vi "CEID Manager.vi"(8 "error in (no error)":errorcluster, 11 "CEID Data":cluster{"CEID":u32, "RPTID":u32[]}[](array[cluster])) -> (0 "error out":errorcluster)   [LabVIEW 2020, in "SECS Scenarios.lvlib" / "34-CEID Setup.lvclass"]
uses:
  34-CEID Setup.lvclass
  SECS Communication/SECS Data Class/CEID Data.ctl
  SECS Communication/SECS Data Class/Remove CEID.vi
  SECS Communication/SECS Data Class/Add CEID.vi
  SECS Communication/SECS Data Class/Get All CEID Data.vi
  SECS Communication/SECS Data Class/SECS Data Class.lvclass
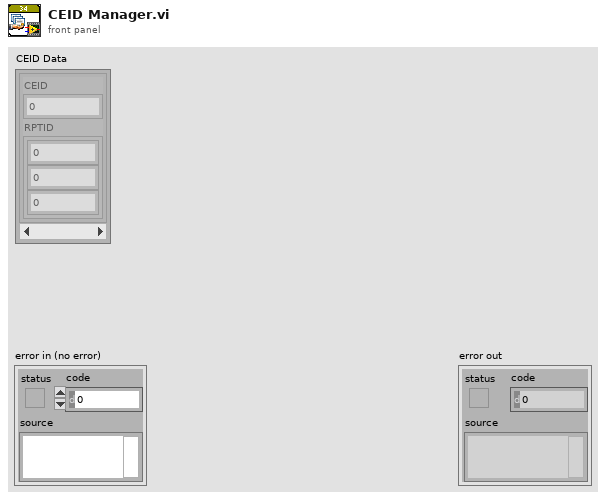
[diagram p1: front panel]
types:
  T1 = typedef "SECS Communication.lvlib/SECS Data Class.lvclass/CEID Data.ctl" = cluster{"Enable":bool, "CEID":u32, "Name":string, "Description":string, "RPTID":u32[], "Dynamic":bool}
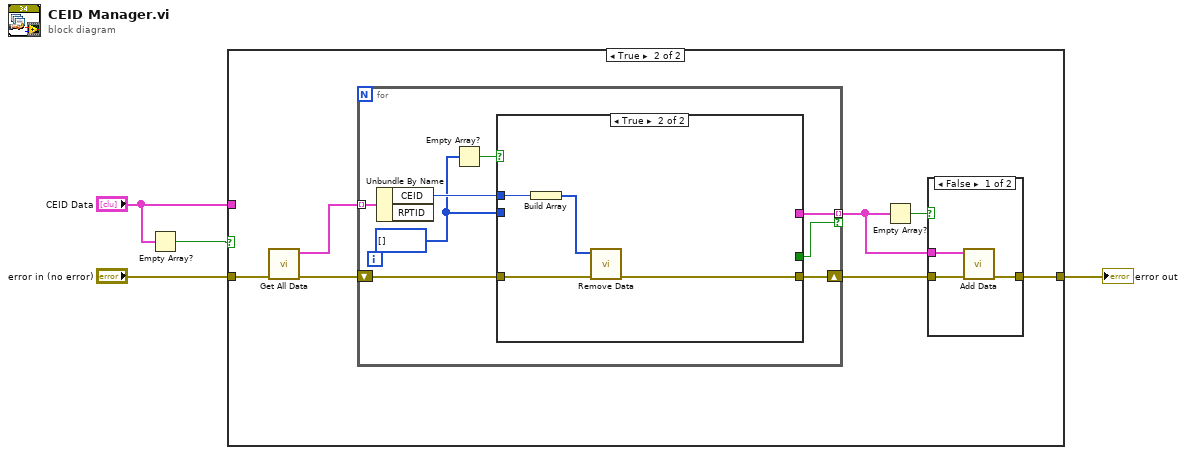
[diagram p0: block diagram]
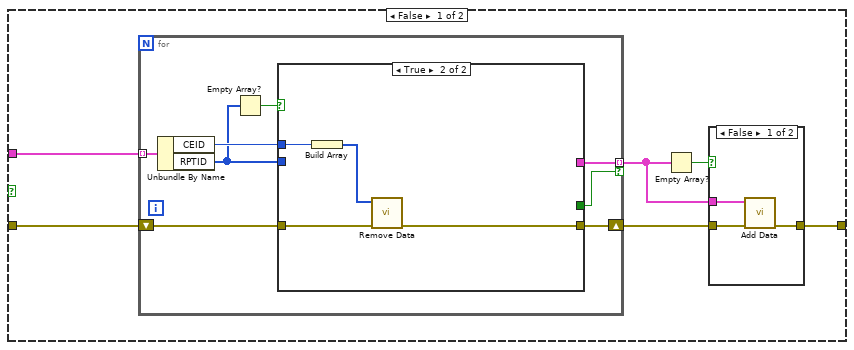
[diagram p2: hidden frame]
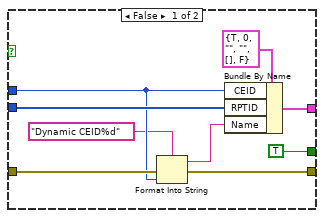
[diagram p4: hidden frame]
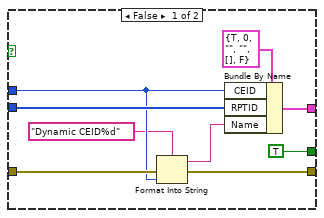
[diagram p6: hidden frame]
diagram:
  n1 = Empty Array?(array="CEID Data") -> (empty?=w1:bool)
  n2 = case shown="True" w1 {
    tunnel: "error in (no error)" -> [w10 w38]
    tunnel: [w9 w42] -> w3
    tunnel: "CEID Data" -> [w5 _]
    frame False {
      n3 = for {
        tunnel: w5 -> [w22] mode=indexing
        shift-right: [w19] -> w8
        shift-left: w10 -> [w20]
        tunnel: [w18] -> w7 mode=indexing if=w15
        n4 = Unbundle By Name(w22) -> ("CEID"=w21:u32, "RPTID"=w17:u32[])
        n5 = Empty Array?(array=w17) -> (empty?=w16:bool)
        n6 = case shown="True" w16 {
          tunnel: w21 -> [w26 w33]
          tunnel: w20 -> [w27 w35]
          tunnel: [w23 w34] -> w19
          tunnel: [w31 _] -> w18
          tunnel: w17 -> [w28 _]
          tunnel: [TRUE _] -> w15
          frame False {
            n7 = Format Into String(format string="Dynamic CEID%d", error in=w27, w26) -> (resulting string=w24:string, error out=w23:errorcluster)  [unwired: 1 in]
            n8 = Bundle By Name(cluster=T1 {"Enable"=TRUE, "CEID"=0, "Name"="", "Description"="", "RPTID"=[], "Dynamic"=FALSE} ("CEID Data In"), "CEID"=w26, "RPTID"=w28, "Name"=w24) -> (w31:T1)
          }
          frame True {
            n9 = Build Array(w33) -> (w32:u32[])
            n10 = call-poly "Remove Data.vi"("error in (no error)"=w35, "CEID"=w32) -> ("error out"=w34:errorcluster)  [unwired: 9 in]
          }
        }
      }
      n11 = Empty Array?(array=w7) -> (empty?=w6:bool)
      n12 = case shown="False" w6 {
        tunnel: [w13 w14] -> w9
        tunnel: w8 -> [w12 w14]
        tunnel: w7 -> [w11 _]
        frame False {
          n13 = call-poly "Add Data.vi"("error in (no error)"=w12, "CEID Data In"=w11) -> ("error out"=w13:errorcluster)  [unwired: 9 in]
        }
        frame True {
        }
      }
    }
    frame True {
      n14 = call-poly "Get All Data.vi"("error in (no error)"=w38) -> ("error out"=w37:errorcluster, "CEID Data"=w36:T1[])  [unwired: 9 in]
      n15 = for {
        tunnel: w36 -> [w54] mode=indexing
        shift-right: [w51] -> w41
        shift-left: w37 -> [w52]
        tunnel: [w50] -> w40 mode=indexing if=w48
        w47 = u32[] [] ("RPTID")
        n16 = Unbundle By Name(w54) -> ("CEID"=w53:u32)  [unwired: 1 out]
        n17 = Empty Array?(array=w47) -> (empty?=w49:bool)
        n18 = case shown="True" w49 {
          tunnel: w53 -> [w58 w65]
          tunnel: w52 -> [w59 w67]
          tunnel: [w55 w66] -> w51
          tunnel: [w63 _] -> w50
          tunnel: w47 -> [w60 _]
          tunnel: [TRUE _] -> w48
          frame False {
            n19 = Format Into String(format string="Dynamic CEID%d", error in=w59, w58) -> (resulting string=w56:string, error out=w55:errorcluster)  [unwired: 1 in]
            n20 = Bundle By Name(cluster=T1 {"Enable"=TRUE, "CEID"=0, "Name"="", "Description"="", "RPTID"=[], "Dynamic"=FALSE} ("CEID Data In"), "CEID"=w58, "RPTID"=w60, "Name"=w56) -> (w63:T1)
          }
          frame True {
            n21 = Build Array(w65) -> (w64:u32[])
            n22 = call-poly "Remove Data.vi"("error in (no error)"=w67, "CEID"=w64) -> ("error out"=w66:errorcluster)  [unwired: 9 in]
          }
        }
      }
      n23 = Empty Array?(array=w40) -> (empty?=w39:bool)
      n24 = case shown="False" w39 {
        tunnel: [w45 w46] -> w42
        tunnel: w41 -> [w44 w46]
        tunnel: w40 -> [w43 _]
        frame False {
          n25 = call-poly "Add Data.vi"("error in (no error)"=w44, "CEID Data In"=w43) -> ("error out"=w45:errorcluster)  [unwired: 9 in]
        }
        frame True {
        }
      }
    }
  }
  "error out" <- w3
